vi "Init Snake.vi"(8 "error in (no error)":errorcluster, 9 "Start Elements":u32, 10 "SnakeColor":u32(colorbox)) -> (0 "error out":errorcluster, 3 "Snake out":refnum<class "Snake.lvclass">)   [LabVIEW 2021, in "Snake.lvclass"]
uses:
  Snake.lvclass
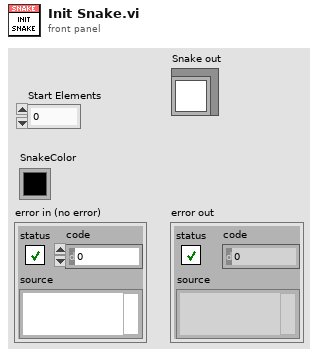
[diagram p1: front panel]
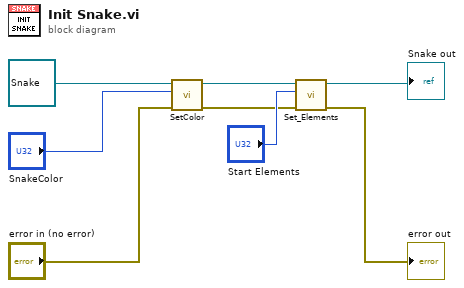
[diagram p0: block diagram]
diagram:
  n1 = call-dynamic "SetColor.vi"("error in (no error)"="error in (no error)", "Color"="SnakeColor", "SnakeGame in"=refnum<class "Snake.lvclass"> refnum ("Snake in")) -> ("error out"=w3:errorcluster, "SnakeGame out"=w5:refnum<class "Snake.lvclass">)  [unwired: 7 in]
  n2 = call-dynamic "Set_Elements.vi"("error in (no error)"=w3, "Start Elements"="Start Elements", "Snake in"=w5) -> ("error out"=→"error out":errorcluster, "Snake out"=→"Snake out":refnum<class "Snake.lvclass">)  [unwired: 7 in]
